vi "Rack.vi"(11 "Full System Configuration":T2={"Rack"=enum."15U; 1-Phase; 16A; 100-240V", "Middle Rail"=enum."None", "Ballast"={"Main"=0, "Small"=0, "Side"=0}, "Front Panel I/O"={"EMO Button"=FALSE, "USB 3.0"=FALSE, "Display"=FALSE, "1st USB 2.0"=FALSE, "2nd USB 2.0"=FALSE, "Ethernet 3"=FALSE, "EMO Extension (3rd Party)"=FALSE, "EMO Extension (Rack In & Out)"=FALSE, "Aux Dual C13 QAC Outlets"=FALSE, "Residual-current Circuit Breaker"=FALSE, "Serial"=FALSE, "GPIB"=FALSE}, "Rear Panel I/O"={"Rear Panel I/O Configuration"=enum."Blank Panel", "EMO Button"=FALSE, "Power, Status & Banana Ground"=FALSE, "Ethernet 2"=FALSE, "Display"=FALSE, "USB 3.0"=FALSE, "DIO"=FALSE, "GPIB"=FALSE, "Aux Dual C13 QAC Outlets"=FALSE, "Residual-current Circuit Breaker"=FALSE, "Serial"=FALSE, "SMA"=FALSE}, "Miscellaneous Options"={"Eyebolts"=FALSE, "Tower Light"=FALSE, "Top/Side Monitor Mount Kit"=FALSE, "24\" Monitor"=FALSE, "Keyboard & Mouse"=FALSE, "Secondary Ethernet Switch"=FALSE, "Extra USB Hub"=FALSE, "USB-6509"=FALSE, "Front Door"=enum."38U (Solid) IG", "Primary Ethernet Switch"=enum."Item 0", "Use Posture"=enum."Item 0"}, "Accessories"={"Screw Type"=enum."10-32", "Cage Nuts & Screws"=0.0, "Filler Panel Color"=enum."Interface Gray", "1U"=0.0, "2U"=0.0, "3U"=0.0}} {"Ballast"."Side" max=5 step=1; "Ballast"."Small" max=5 step=1; "Ballast"."Main" max=5 step=1}) -> (3 "cluster":T1)   [LabVIEW 2023]
uses:
  Option Type Defs/Full System Configuration.ctl
  Option Type Defs/Rack.ctl
  Option Type Defs/Middle Rail.ctl
  Option Type Defs/Ballast.ctl
  Option Type Defs/Front Panel IO.ctl
  Option Type Defs/Rear Panel IO.ctl
  Option Type Defs/Rear Panel IO Configuration.ctl
  Option Type Defs/Miscellaneous Options.ctl
  Option Type Defs/Front Door.ctl
  Option Type Defs/Parts List.ctl
  <userlib>/_OpenG.lib/lvdata/lvdata.llb/openg_variant.lvlib
  Option Type Defs/Screw Types.ctl
  Option Type Defs/Filler Panel Color.ctl
  Option Type Defs/Accessories.ctl
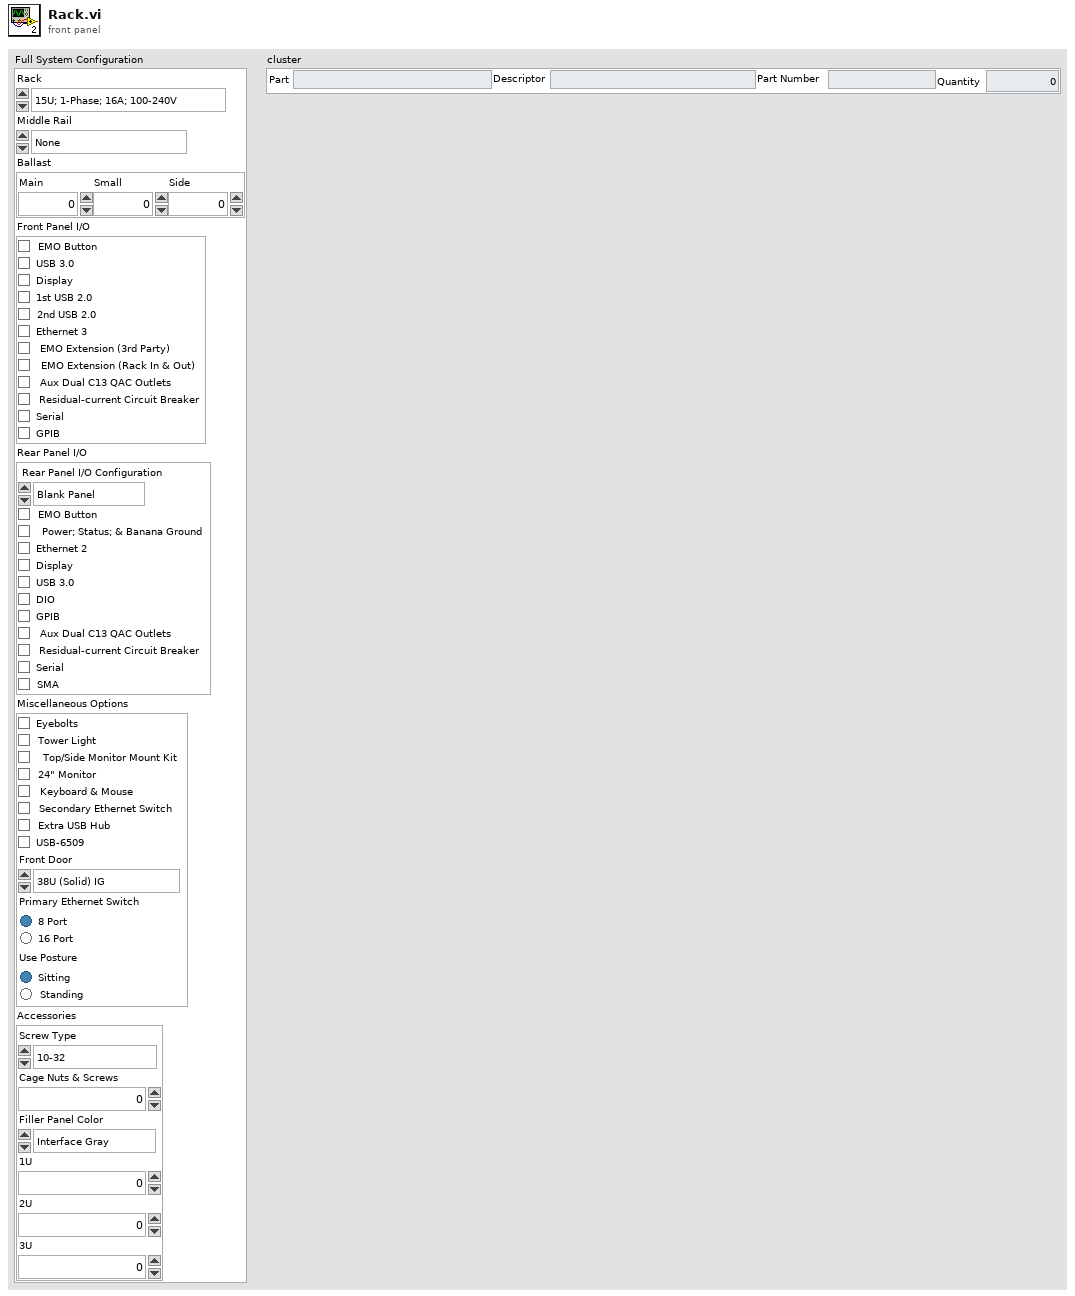
[diagram p1: front panel]
types:
  T1 = typedef "Parts List.ctl" = cluster{"Part":string, "Descriptor":string, "Part Number":string, "Quantity":dbl}
  T2 = typedef "Full System Configuration.ctl" = cluster{"Rack":T3, "Middle Rail":T4, "Ballast":T5, "Front Panel I/O":T6, "Rear Panel I/O":T7, "Miscellaneous Options":T9, "Accessories":T11}
  T3 = typedef "Rack.ctl" = enum16{"15U; 1-Phase; 16A; 100-240V", "15U; 1-Phase; 24A; 100-240V", "38U; 3-Phase Delta; 50A; 200-240V", "38U; 1-Phase; 24A; 100-120V", "38U; 3-Phase Wye; 50A; 200-240V", "38U; 3-Phase Delta; 50A; 380-480V", "38U; 3-Phase Delta; 32A; 200-240V", "38U; 3-Phase Wye; 16A; 100-240V", "44U; 1-Phase; 24A; 100-240V", "44U; 3-Phase Delta; 32A; 200-240V"}
  T4 = typedef "Middle Rail.ctl" = enum16{"None", "Flip Side Rear; D=168.83mm", "Parallel Rear; D=145mm", "Flip Side Front; D=145mm", "Parallel Front; D=145mm"}
  T5 = typedef "Ballast.ctl" = cluster{"Main":u16, "Small":u16, "Side":u16}
  T6 = typedef "Front Panel IO.ctl" = cluster{"EMO Button":bool, "USB 3.0":bool, "Display":bool, "1st USB 2.0":bool, "2nd USB 2.0":bool, "Ethernet 3":bool, "EMO Extension (3rd Party)":bool, "EMO Extension (Rack In & Out)":bool, "Aux Dual C13 QAC Outlets":bool, "Residual-current Circuit Breaker":bool, "Serial":bool, "GPIB":bool}
  T7 = typedef "Rear Panel IO.ctl" = cluster{"Rear Panel I/O Configuration":T8, "EMO Button":bool, "Power, Status & Banana Ground":bool, "Ethernet 2":bool, "Display":bool, "USB 3.0":bool, "DIO":bool, "GPIB":bool, "Aux Dual C13 QAC Outlets":bool, "Residual-current Circuit Breaker":bool, "Serial":bool, "SMA":bool}
  T8 = typedef "Rear Panel IO Configuration.ctl" = enum16{"Blank Panel", "Fully Populated Panel", "Custom Panel"}
  T9 = typedef "Miscellaneous Options.ctl" = cluster{"Eyebolts":bool, "Tower Light":bool, "Top/Side Monitor Mount Kit":bool, "24\" Monitor":bool, "Keyboard & Mouse":bool, "Secondary Ethernet Switch":bool, "Extra USB Hub":bool, "USB-6509":bool, "Front Door":T10, "Primary Ethernet Switch":enum32{"Item 0", "Item 1"}, "Use Posture":enum32{"Item 0", "Item 1"}}
  T10 = typedef "Front Door.ctl" = enum16{"None", "38U (Solid) IG", "38U (Solid) EG", "38U: Top 14U (Solid) IG", "38U (Clear) IG", "44U (Solid) IG", "44U (Solid) EG"}
  T11 = typedef "Accessories.ctl" = cluster{"Screw Type":T12, "Cage Nuts & Screws":dbl, "Filler Panel Color":T13, "1U":dbl, "2U":dbl, "3U":dbl}
  T12 = typedef "Screw Types.ctl" = enum16{"None", "M6 (Most Common)", "10-32", "12-24"}
  T13 = typedef "Filler Panel Color.ctl" = enum16{"None", "Interface Gray", "Environmental Gray"}
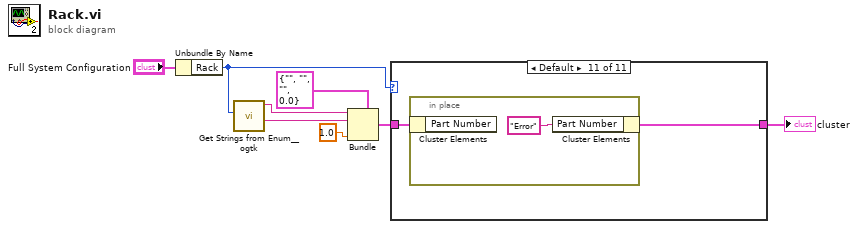
[diagram p0: block diagram]
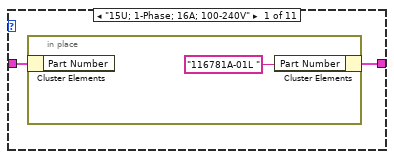
[diagram p2: hidden frame]
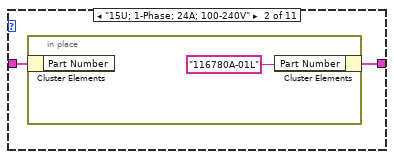
[diagram p3: hidden frame]
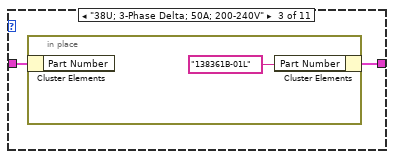
[diagram p4: hidden frame]
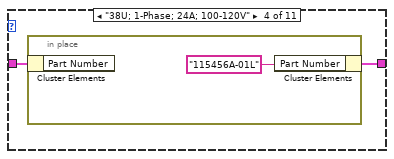
[diagram p5: hidden frame]
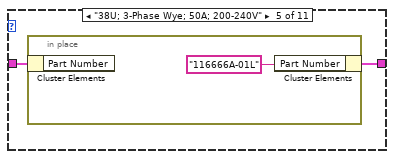
[diagram p6: hidden frame]
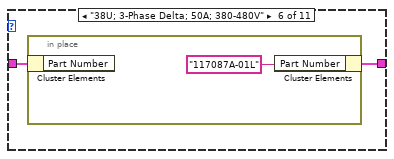
[diagram p7: hidden frame]
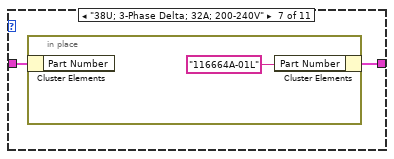
[diagram p8: hidden frame]
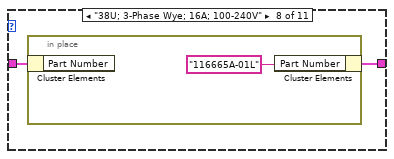
[diagram p9: hidden frame]
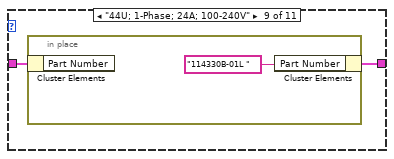
[diagram p10: hidden frame]
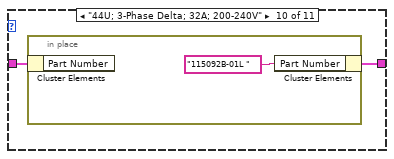
[diagram p11: hidden frame]
diagram:
  n1 = Unbundle By Name("Full System Configuration") -> ("Rack"=w8:T3)
  n2 = call <userlib>:"Get Strings from Enum__ogtk.vi"("Enum"=w8) -> ("String Value"=w2:string, "Enum Name"=w3:string)  [unwired: 7 in, 2 out]
  n3 = Bundle(cluster=T1 {"Part"="", "Descriptor"="", "Part Number"="", "Quantity"=0.0}, "Part"=w3, "Descriptor"=w2, "Quantity"=1.0) -> (w5:T1)  [unwired: 1 in]
  n4 = case shown="Default" w8 {
    tunnel: w5 -> [w10 w13 w16 w19 w22 w25 w28 w31 w34 w37 w40]
    tunnel: [w9 w12 w15 w18 w21 w24 w27 w30 w33 w36 w39] -> w6
    frame "15U; 1-Phase; 16A; 100-240V" {
      n5 = in-place {
        n6 = in-place-cluster #1(w10) -> ()  [unwired: 1 out]
        n7 = in-place-cluster #1("Part Number"="116781A-01L ") -> (w9:T1)
      }
    }
    frame "15U; 1-Phase; 24A; 100-240V" {
      n8 = in-place {
        n9 = in-place-cluster #2(w13) -> ()  [unwired: 1 out]
        n10 = in-place-cluster #2("Part Number"="116780A-01L") -> (w12:T1)
      }
    }
    frame "38U; 3-Phase Delta; 50A; 200-240V" {
      n11 = in-place {
        n12 = in-place-cluster #3(w16) -> ()  [unwired: 1 out]
        n13 = in-place-cluster #3("Part Number"="138361B-01L") -> (w15:T1)
      }
    }
    frame "38U; 1-Phase; 24A; 100-120V" {
      n14 = in-place {
        n15 = in-place-cluster #4(w19) -> ()  [unwired: 1 out]
        n16 = in-place-cluster #4("Part Number"="115456A-01L") -> (w18:T1)
      }
    }
    frame "38U; 3-Phase Wye; 50A; 200-240V" {
      n17 = in-place {
        n18 = in-place-cluster #5(w22) -> ()  [unwired: 1 out]
        n19 = in-place-cluster #5("Part Number"="116666A-01L") -> (w21:T1)
      }
    }
    frame "38U; 3-Phase Delta; 50A; 380-480V" {
      n20 = in-place {
        n21 = in-place-cluster #6(w25) -> ()  [unwired: 1 out]
        n22 = in-place-cluster #6("Part Number"="117087A-01L") -> (w24:T1)
      }
    }
    frame "38U; 3-Phase Delta; 32A; 200-240V" {
      n23 = in-place {
        n24 = in-place-cluster #7(w28) -> ()  [unwired: 1 out]
        n25 = in-place-cluster #7("Part Number"="116664A-01L") -> (w27:T1)
      }
    }
    frame "38U; 3-Phase Wye; 16A; 100-240V" {
      n26 = in-place {
        n27 = in-place-cluster #8(w31) -> ()  [unwired: 1 out]
        n28 = in-place-cluster #8("Part Number"="116665A-01L") -> (w30:T1)
      }
    }
    frame "44U; 1-Phase; 24A; 100-240V" {
      n29 = in-place {
        n30 = in-place-cluster #9(w34) -> ()  [unwired: 1 out]
        n31 = in-place-cluster #9("Part Number"="114330B-01L ") -> (w33:T1)
      }
    }
    frame "44U; 3-Phase Delta; 32A; 200-240V" {
      n32 = in-place {
        n33 = in-place-cluster #10(w37) -> ()  [unwired: 1 out]
        n34 = in-place-cluster #10("Part Number"="115092B-01L ") -> (w36:T1)
      }
    }
    frame Default {
      n35 = in-place {
        n36 = in-place-cluster #11(w40) -> ()  [unwired: 1 out]
        n37 = in-place-cluster #11("Part Number"="Error") -> (w39:T1)
      }
    }
  }
  "cluster" <- w6
